vi "Get SQL formatted value.vi"(8 "error in (no error)":errorcluster, 11 "String Column in":refnum<class "String Column.lvclass">) -> (0 "error out":errorcluster, 2 "Formatted Value":string, 3 "String Column out":refnum<class "String Column.lvclass">)   [LabVIEW 2020, in "Basic Columns.lvlib" / "String Column.lvclass"]
uses:
  String Column.lvclass
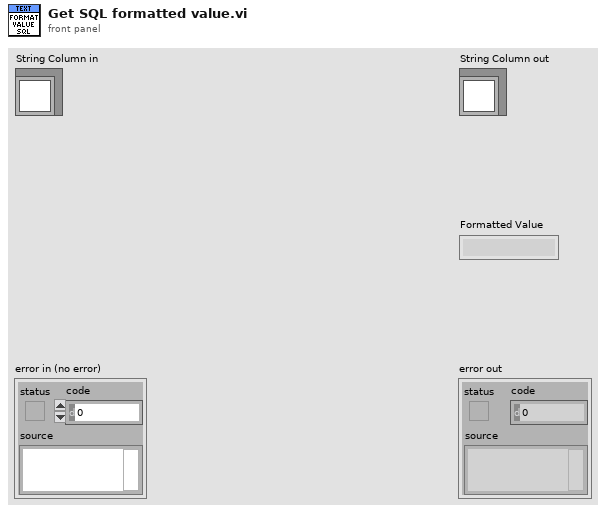
[diagram p1: front panel]
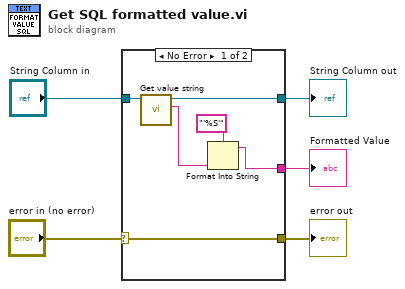
[diagram p0: block diagram]
diagram:
  n1 = case shown="No Error" "error in (no error)" {
    selector: "error in (no error)" -> [w7 w13]
    tunnel: [w7 w13] -> w4
    tunnel: "String Column in" -> [w11 w12]
    tunnel: [w10 w12] -> w2
    tunnel: [w8 _] -> w1
    frame No Error {
      n2 = call-dynamic "Get value string.vi"("Column in"=w11) -> ("Value"=w6:string, "Column out"=w10:refnum<class "String Column.lvclass">)  [unwired: 8 in, 1 out]
      n3 = Format Into String(format string="'%S'", w6) -> (resulting string=w8:string)  [unwired: 2 in, 1 out]
    }
    frame Error {
    }
  }
  "error out" <- w4
  "String Column out" <- w2
  "Formatted Value" <- w1
